vi "freqread.vi"() -> ()   [LabVIEW 2015]
uses:
  <vilib>/Utility/file.llb/Write Delimited Spreadsheet (string).vi
panel:
  out "Waveform Chart":dynamicdata(graph)
  out "Microwave Frequency":dbl format="%#.6g"
  out "error out":errorcluster
  in  "error in (no error)":errorcluster
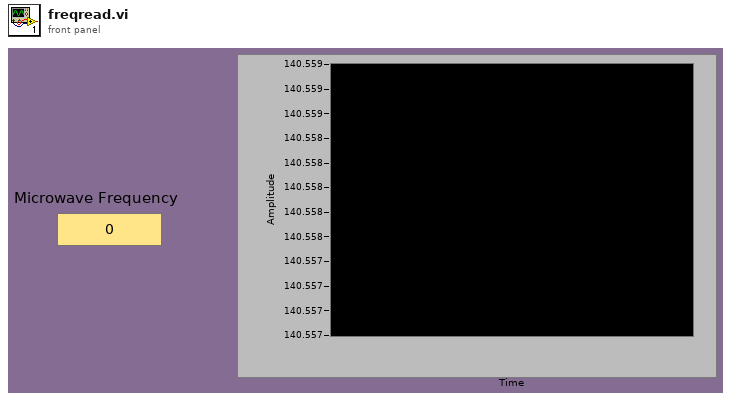
[diagram p1: front panel]
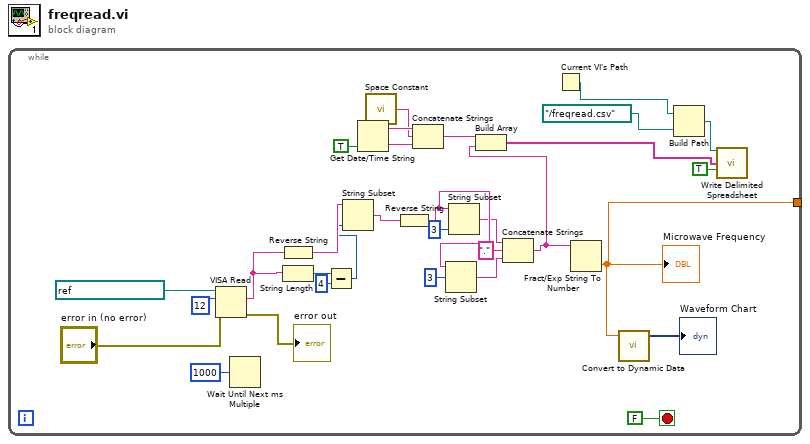
[diagram p0: block diagram]
diagram:
  n1 = while {
    tunnel: [w1] -> _
    stop <- FALSE stop-if-true
    n2 = VISA Read(VISA resource name=refnum<visa-resource-name> "GPIB0::3::INSTR", byte count=u32 12, error in (no error)="error in (no error)") -> (read buffer=w26:string, error out=→"error out":errorcluster)  [unwired: 2 out]
    n3 = Wait Until Next ms Multiple(millisecond multiple=u32 1000) -> ()  [unwired: 1 out]
    n4 = Reverse String(1:w26) -> (0:w23:string)
    n5 = String Length(string=w26) -> (length=w25:i32)
    n6 = Subtract(x=w25, y=4) -> (x-y=w22:i32)
    n7 = String Subset(string=w23, length (rest)=w22) -> (substring=w21:string)  [unwired: 1 in]
    n8 = Get Date/Time String(want seconds? (F)=TRUE) -> (date string=w11:string, time string=w9:string)  [unwired: 2 in]
    n9 = call <vilib>:"Space Constant.vi"() -> ("String"=w10:string)
    n10 = Reverse String(1:w21) -> (0:w19:string)
    n11 = Concatenate Strings(w11, w10, w9) -> (w8:string)
    n12 = String Subset(string=w19, offset (0)=3) -> (substring=w17:string)  [unwired: 1 in]
    n13 = String Subset(string=w19, length (rest)=3 ("length (rest)")) -> (substring=w16:string)  [unwired: 1 in]
    n14 = Concatenate Strings(w16, "." ("string"), w17) -> (w7:string)
    n15 = Build Array(w8, w7) -> (w4:string[])
    n16 = Current VI's Path() -> (path=w3:path)
    n17 = Fract/Exp String To Number(string=w7) -> (number=w1:dbl)  [unwired: 3 in, 1 out]
    "Microwave Frequency" <- w1
    n18 = call "Convert to Dynamic Data"("Double"=w1) -> ("Dynamic Data Type"=→"Waveform Chart":dynamicdata)  [unwired: 3 in]
    n19 = Build Path(base path=w3, name or relative path=path "../freqread.csv" ("base path")) -> (appended path=w5:path)
    n20 = call-poly <vilib>:"Write Delimited Spreadsheet.vi"("file path (dialog if empty)"=w5, "1D data"=w4, "append to file? (F)"=TRUE) -> ()  [unwired: 11 in, 2 out]
  }
